vi "Begin.vi"(8 "error in":errorcluster) -> (0 "error out":errorcluster)   [LabVIEW 2014]
doc: "Called before other user functions, this VI is expected to open initial I/O refnums, load in file data, and do all program initialization. Notice that the <B>error out</B> terminal is simply used for data flow. Wiring it to other structures or subVIs ensures that this VI runs first."
uses:
  <vilib>/Rock Robotics/WPI/DriverStation/WPI_DriverStationRobotMode2.ctl
  <vilib>/Rock Robotics/WPI/Joystick/WPI_JoystickDeviceEnum.ctl
  <vilib>/Rock Robotics/SystemInterfaces/DIO/FPGA_DIOPWMChannel.ctl
  <vilib>/Rock Robotics/WPI/SafetyOutput/WPI_SafetyOutputConfigMenu.ctl
  Robot Global Data.vi
  <vilib>/Rock Robotics/Network Tables/SD Write String Array.vi
  <vilib>/Rock Robotics/WPI/Compressor/WPI_CompressorGetSetRefNum.vi
  <vilib>/Rock Robotics/WPI/RobotDrive/WPI_RobotDriveOpen4MotorWithVictor.vi
  <vilib>/Rock Robotics/WPI/MotorControl/WPI_MotorControlOpen Talon.vi
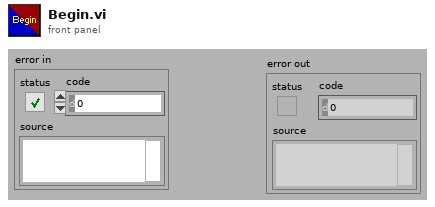
[diagram p1: front panel]
types:
  T1 = typedef "WPI_SafetyOutputConfigMenu.ctl" = enum16{"Enable", "Disable"}
  T2 = typedef "FPGA_DIOPWMChannel.ctl" = enum8{"PWM 0", "PWM 1", "PWM 2", "PWM 3", "PWM 4", "PWM 5", "PWM 6", "PWM 7", "PWM 8", "PWM 9", "PWM MXP 0", "PWM MXP 1", "PWM MXP 2", "PWM MXP 3", "PWM MXP 4", "PWM MXP 5", "PWM MXP 6", "PWM MXP 7", "PWM MXP 8", "PWM MXP 9", "Invalid"}
  T3 = typedef "WPI_JoystickDeviceEnum.ctl" = enum16{"USB 0", "USB 1", "USB 2", "USB 3", "USB 4", "USB 5"}
  T4 = typedef "WPI_DriverStationRobotMode2.ctl" = enum16{"Autonomous Disabled", "Autonomous Enabled", "Teleop Disabled", "Teleop Enabled", "Disconnected", "Finish", "Test Disabled", "Test Enabled", "Emergency Stopped"}
  T5 = typedef "WPI_RobotDriveDevRef.ctl" = cluster{"DevStatus":errorcluster, "Motors[]":T6[], "Square Inputs":bool, "Max Output":dbl}
  T6 = typedef "WPI_MotorControlDeviceRef.ctl" = cluster{"DeviceStatus":errorcluster, "Type":T7, "PWM":cluster{"Controller":T8, "PWM Channel":T2, "DeadBand":T9}, "CAN":cluster{"Device Number":u8, "Control Mode":T10, "Semaphore":T11, "Max Vout":dbl, "TalonSRX Control Mode":T12}, "Invert":bool, "TransformRef":T13, "InvTransformRef":T13}
  T7 = typedef "WPI_MotorControlType.ctl" = enum16{"PWM", "CAN", "CANTalonSRX"}
  T8 = typedef "FPGA_TypedefDigitalModule.ctl" = enum16{"Controller 1"}
  T9 = typedef "WPI_PWMDeadband.ctl" = cluster{"Name":string, "maxPositivePwm":i32, "minPositivePwm":i32, "centerPwm":i32, "maxNegativePwm":i32, "minNegativePwm":i32, "angularRange":u16}
  T10 = typedef "WPI_CANJaguar_ControlMode.ctl" = enum8{"Percent VBus", "Current", "Speed", "Position", "Voltage"}
  T11 = typedef "Semaphore RefNum" = refnum<k1>
  T12 = typedef "WPI_CANTalonSRX_APIControlMode.ctl" = enum8{"Percent VBus", "Speed", "Position", "Slave", "Unchanged / Invalid"}
  T13 = typedef "WPI_PWMTransform_ConPane.ctl" = refnum<vi>
  T14 = typedef "WPI_JoystickDevRef.ctl" = cluster{"Device":T3}
  T15 = typedef "WPI_CompressorDevRef.ctl" = cluster{"DevStatus":errorcluster, "Pneumatics Control Module":u8}
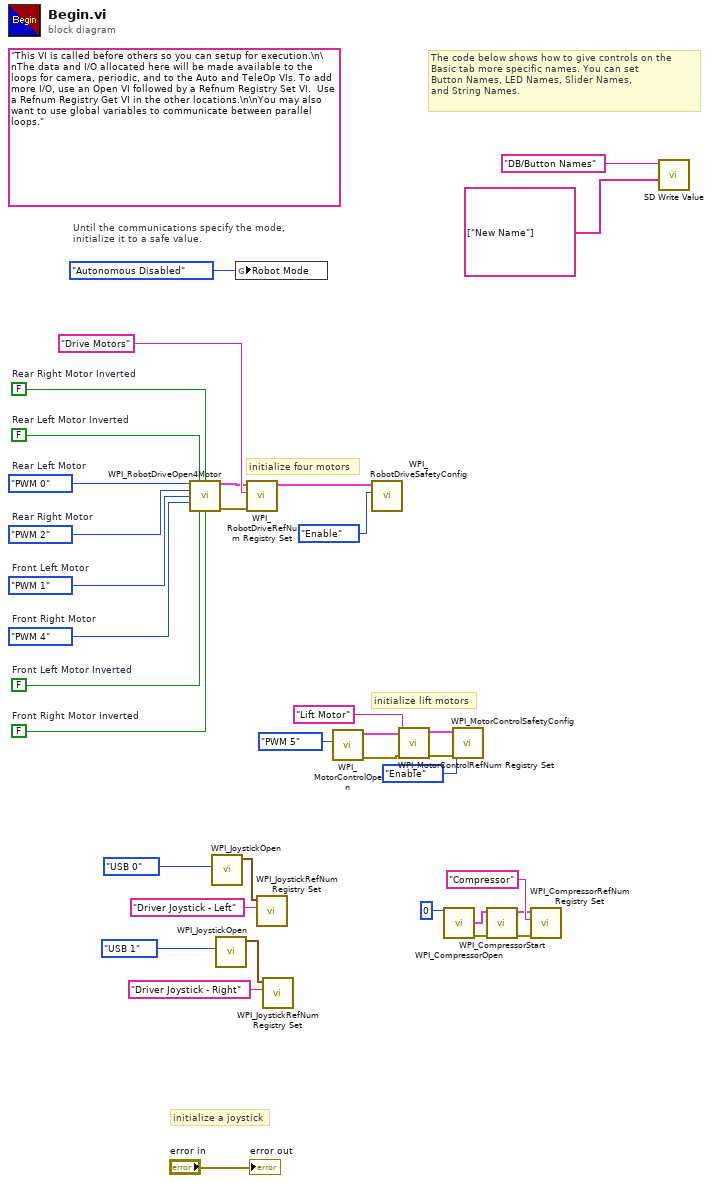
[diagram p0: block diagram]
diagram:
  w8 = FPGA_DIOPWMChannel."PWM 4"  # Front Right Motor
  w9 = FPGA_DIOPWMChannel."PWM 1"  # Front Left Motor
  w10 = FPGA_DIOPWMChannel."PWM 2"  # Rear Right Motor
  w11 = FPGA_DIOPWMChannel."PWM 0"  # Rear Left Motor
  w12 = FALSE  # Front Left Motor Inverted
  w13 = FALSE  # Front Right Motor Inverted
  w14 = FALSE  # Rear Left Motor Inverted
  w15 = FALSE  # Rear Right Motor Inverted
  (unwired) "This VI is called before others so you can setup for execution.\n\nThe data and I/O allocated here will be made available to the loops for camera, periodic, and to the Auto and TeleOp VIs. To add more I/O, use an Open VI followed by a Refnum Registry Set VI.  Use a Refnum Registry Get VI in the other locations.\n\nYou may also want to use global variables to communicate between parallel loops."
  # "initialize lift motors"
  # "The code below shows how to give controls on the\nBasic tab more specific names. You can set\nButton Names, LED Names, Slider Names,\nand String Names."
  # "initialize a joystick"
  # "Until the communications specify the mode,\ninitialize it to a safe value."
  # "initialize four motors"
  n1 = call-poly <vilib>:"WPI_RobotDriveOpen4Motor.vi"("Rear Left Motor"=w11, "Rear Left Motor Inverted"=w14, "Rear Right Motor Inverted"=w15, "Rear Right Motor"=w10, "Front Left Motor"=w9, "Front Right Motor"=w8, "Front Left Motor Inverted"=w12, "Front Right Motor Inverted"=w13) -> ("RobotDriveDevRef"=w17:T5, "error out"=w16:errorcluster)  [unwired: 6 in]
  n2 = call <vilib>:"WPI_JoystickOpen.vi"("JoystickDevice"=WPI_JoystickDeviceEnum."USB 0") -> ("JoystickDevRef"=w31:T14)  [unwired: 10 in]
  n3 = call <vilib>:"WPI_JoystickOpen.vi"("JoystickDevice"=WPI_JoystickDeviceEnum."USB 1") -> ("JoystickDevRef"=w25:T14)  [unwired: 10 in]
  n4 = global write "Robot Global Data.vi" "Robot Mode"(WPI_DriverStationRobotMode2."Autonomous Disabled" ("Robot Mode")) -> ()
  n5 = call <vilib>:"WPI_RobotDriveRefNum Registry Set.vi"("error in (no error)"=w16, "refnum name"="Drive Motors", "RobotDriveDevRef"=w17) -> ("RobotDriveDevRef"=w35:T5)  [unwired: 8 out]
  n6 = call <vilib>:"WPI_JoystickRefNum Registry Set.vi"("refnum name"="Driver Joystick - Left", "JoystickDevRef"=w31) -> ()  [unwired: 8 in, 2 out]
  n7 = call <vilib>:"WPI_JoystickRefNum Registry Set.vi"("refnum name"="Driver Joystick - Right", "JoystickDevRef"=w25) -> ()  [unwired: 8 in, 2 out]
  n8 = call-poly <vilib>:"WPI_MotorControlOpen.vi"("PWM Channel"=FPGA_DIOPWMChannel."PWM 5") -> ("error out"=w6:errorcluster, "MotorControlDeviceRef"=w7:T6)  [unwired: 9 in]
  n9 = call <vilib>:"WPI_RobotDriveSafetyConfig.vi"("mode"=WPI_SafetyOutputConfigMenu."Enable", "RobotDriveDevRef"=w35) -> ()  [unwired: 8 in, 2 out]
  n10 = call <vilib>:"WPI_MotorControlRefNum Registry Set.vi"("error in (no error)"=w6, "refnum name"="Lift Motor", "MotorControlDevRef"=w7) -> ("error out"=w5:errorcluster, "MotorControlDevRef"=w4:T6)  [unwired: 7 in]
  n11 = call <vilib>:"WPI_CompressorOpen.vi"("Pneumatics Control Module (0)"=u8 0) -> ("CompressorDevRef"=w20:T15, "error out"=w21:errorcluster)  [unwired: 13 in]
  n12 = call <vilib>:"WPI_MotorControlSafetyConfig.vi"("error in (no error)"=w5, "mode"=WPI_SafetyOutputConfigMenu."Enable", "MotorControlDevRef"=w4) -> ()  [unwired: 7 in, 2 out]
  n13 = call <vilib>:"WPI_CompressorStart.vi"("error in (no error)"=w21, "CompressorDevRef"=w20) -> ("error out"=w19:errorcluster, "CompressorDevRef"=w18:T15)  [unwired: 8 in]
  n14 = call <vilib>:"WPI_CompressorRefNum Registry Set.vi"("error in (no error)"=w19, "refnum name"="Compressor", "CompressorDevRef"=w18) -> ()  [unwired: 7 in, 2 out]
  n15 = call-poly <vilib>:"SD Write Value.vi"("String Array"=string[] ["New Name"], "Name"="DB/Button Names") -> ()  [unwired: 8 in, 2 out]
  "error out" <- "error in"
